vi "Build from database.vi"(8 "error in (no error)":errorcluster, 10 "Table Configuration":refnum<class "Table Configuration Interface.lvclass">, 11 "Table in":refnum<class "Basic Table.lvclass">) -> (0 "error out":errorcluster, 3 "Table out":refnum<class "Basic Table.lvclass">)   [LabVIEW 2020, in "Table.lvlib" / "Basic Table.lvclass"]
uses:
  Basic Table.lvclass
  Table Configuration Interface/Table Configuration Interface.lvclass
  Basic Table.lvclass/Basic Table.ctl
  Database Libraries/Database Interfaces/Primary Key Info.ctl
  Column Libraries/Basic Columns/Column Configuration/Basic Column Configuration Class/Column Configuration.lvclass
  Database Libraries/Database Interfaces/Database Interface Class/Database Interface.lvclass
  Column Libraries/Basic Columns/Column Configuration/Column Factory Parent Class/Column Factory.lvclass
  Database Libraries/Database Interfaces.lvlib
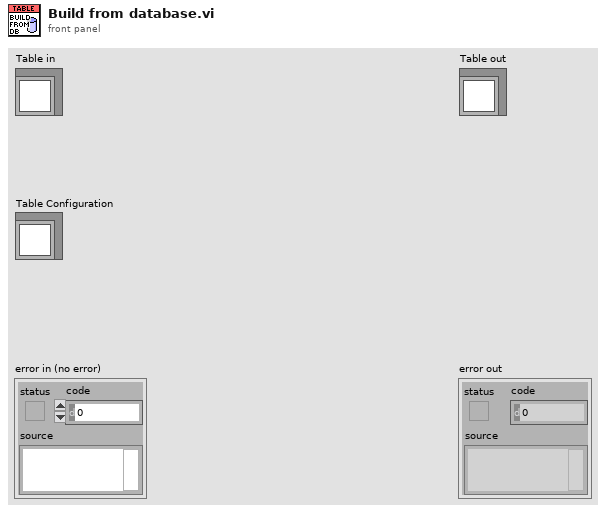
[diagram p1: front panel]
types:
  T1 = typedef "Database Interfaces.lvlib/Primary Key Info.ctl" = cluster{"Primary Key Column":string, "Display Column":string}
  T2 = typedef "Column Interfaces.lvlib/FK Info.ctl" = cluster{"PK Table":string, "PK Column":string, "PK Display Column":string}
  T3 = typedef "Database Interfaces.lvlib/Column Information.ctl" = cluster{"Name":string, "Type":T4, "Size (bytes)":i32}
  T4 = typedef "Database Interfaces.lvlib/Database data type.ctl" = enum16{"Undefined", "String", "Long (I32)", "Single (SGL)", "Double (DBL)", "Date/Time", "Binary"}
  T5 = map{string, refnum<class "Column Interface.lvclass">}
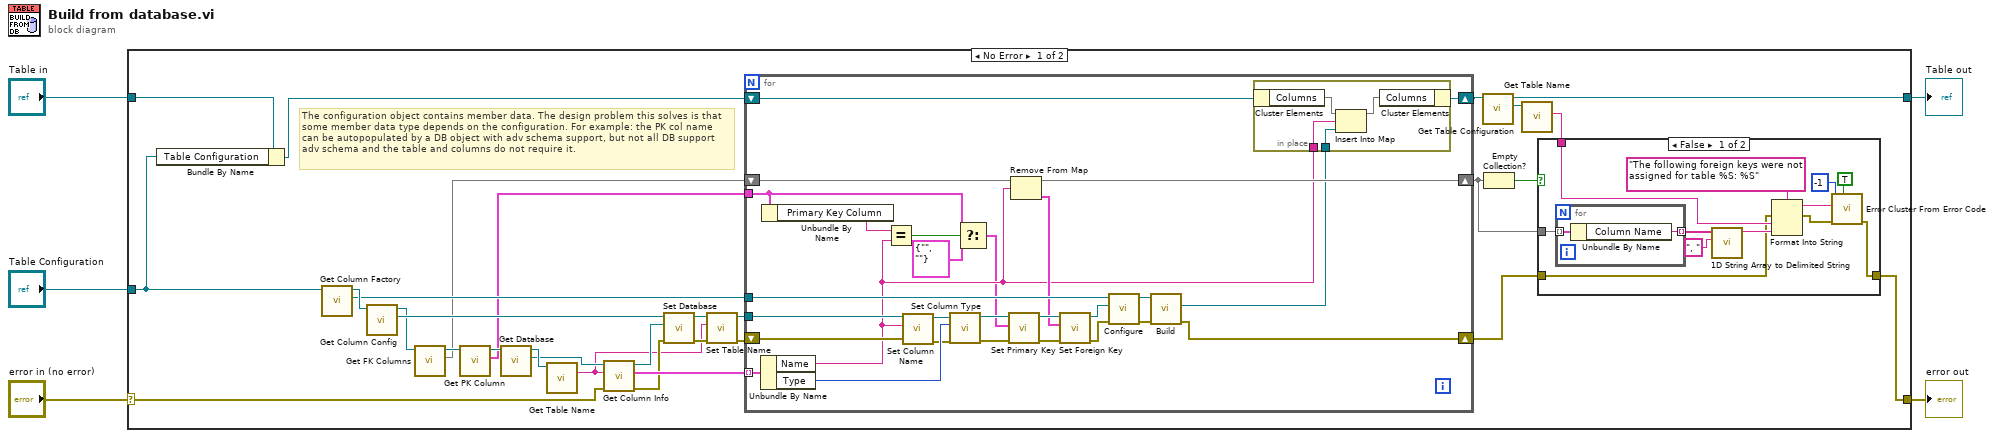
[diagram p0: block diagram]
diagram:
  n1 = case shown="No Error" "error in (no error)" {
    selector: "error in (no error)" -> [w29 w84]
    tunnel: [w7 w84] -> w4
    tunnel: [w10 w83] -> w2
    tunnel: "Table in" -> [w21 w83]
    tunnel: "Table Configuration" -> [w19 _]
    frame No Error {
      # "The configuration object contains member data. The design problem this solves is that some member data type depends on the configuration. For example: the PK col name can be autopopulated by a DB object with adv schema support, but not all DB support adv schema and the table and columns do not require it."
      n2 = Bundle By Name(cluster=w21, "Table Configuration"=w19) -> (w20:refnum<class "Basic Table.lvclass">)
      n3 = call-dynamic "Get Column Factory.vi"("Table Configuration Interface in"=w19) -> ("Column Factory"=w25:refnum<class "Column Factory.lvclass">, "Table Configuration Interface out"=w27:refnum<class "Table Configuration Interface.lvclass">)  [unwired: 8 in, 1 out]
      n4 = call-dynamic "Get Column Config.vi"("Table Configuration Interface in"=w27) -> ("Column Configuration"=w24:refnum<class "Column Configuration.lvclass">, "Table Configuration Interface out"=w18:refnum<class "Table Configuration Interface.lvclass">)  [unwired: 8 in, 1 out]
      n5 = call-dynamic "Get FK Columns.vi"("Table Configuration Interface in"=w18) -> ("FKs"=w15:map{string, T2}, "Table Configuration Interface out"=w17:refnum<class "Table Configuration Interface.lvclass">)  [unwired: 8 in, 1 out]
      n6 = call-dynamic "Get PK Column.vi"("Table Configuration Interface in"=w17) -> ("Primary Key"=w6:T1, "Table Configuration Interface out"=w16:refnum<class "Table Configuration Interface.lvclass">)  [unwired: 8 in, 1 out]
      n7 = call-dynamic "Get Database.vi"("Table Configuration Interface in"=w16) -> ("Database"=w23:refnum<class "Database Interface.lvclass">, "Table Configuration Interface out"=w26:refnum<class "Table Configuration Interface.lvclass">)  [unwired: 8 in, 1 out]
      n8 = call-dynamic "Get Table Name.vi"("Table Configuration Interface in"=w26) -> ("Table Name"=w22:string)  [unwired: 8 in, 2 out]
      n9 = call-dynamic "Get Column Info.vi"("error in (no error)"=w29, "Table Name"=w22, "Database Interface in"=w23) -> ("error out"=w32:errorcluster, "Column Information Array"=w35:T3[], "Database Interface out"=w28:refnum<class "Database Interface.lvclass">)  [unwired: 6 in]
      n10 = call-dynamic "Set Database.vi"("error in (no error)"=w32, "Database"=w28, "Basic Column Configuration in"=w24) -> ("error out"=w31:errorcluster, "Basic Column Configuration out"=w34:refnum<class "Column Configuration.lvclass">)  [unwired: 7 in]
      n11 = call-dynamic "Set Table Name.vi"("error in (no error)"=w31, "Table Name"=w22, "Basic Column Configuration in"=w34) -> ("error out"=w30:errorcluster, "Basic Column Configuration out"=w33:refnum<class "Column Configuration.lvclass">)  [unwired: 7 in]
      n12 = for {
        tunnel: w35 -> [w78] mode=indexing
        tunnel: w33 -> [w76]
        tunnel: w25 -> [w74]
        shift-right: [w71] -> w11
        shift-left: w20 -> [w72]
        shift-right: [w67] -> w12
        shift-left: w30 -> [w70]
        shift-right: [w59] -> w13
        shift-left: w15 -> [w60]
        tunnel: w6 -> [w55]
        n13 = Unbundle By Name(w78) -> ("Name"=w57:string, "Type"=w77:T4)
        n14 = Unbundle By Name(w55) -> ("Primary Key Column"=w56:string)
        n15 = Equal?(x=w56, y=w57) -> (x = y?=w52:bool)
        n16 = call-dynamic "Set Column Name.vi"("error in (no error)"=w70, "Column Name"=w57, "Basic Column Configuration in"=w76) -> ("error out"=w69:errorcluster, "Basic Column Configuration out"=w75:refnum<class "Column Configuration.lvclass">)  [unwired: 7 in]
        n17 = call-dynamic "Set Column Type.vi"("error in (no error)"=w69, "Column Type"=w77, "Basic Column Configuration in"=w75) -> ("error out"=w65:errorcluster, "Basic Column Configuration out"=w66:refnum<class "Column Configuration.lvclass">)  [unwired: 7 in]
        n18 = Select(t=w55, s=w52, f=T1 {"Primary Key Column"="", "Display Column"=""}) -> (s? t:f=w53:T1)
        n19 = call-dynamic "Set Primary Key.vi"("error in (no error)"=w65, "Primary Key"=w53, "Basic Column Configuration in"=w66) -> ("error out"=w63:errorcluster, "Basic Column Configuration out"=w64:refnum<class "Column Configuration.lvclass">)  [unwired: 7 in]
        n20 = Remove From Map(10:w57, 11:w60) -> (1:w58:T2, 3:w59:map{string, T2})  [unwired: 1 out]
        n21 = call-dynamic "Set Foreign Key.vi"("error in (no error)"=w63, "FK Info"=w58, "Basic Column Configuration in"=w64) -> ("error out"=w62:errorcluster, "Basic Column Configuration out"=w61:refnum<class "Column Configuration.lvclass">)  [unwired: 7 in]
        n22 = call-dynamic "Configure.vi"("error in (no error)"=w62, "Configuration"=w61, "Column Factory in"=w74) -> ("error out"=w68:errorcluster, "Column Factory out"=w73:refnum<class "Column Factory.lvclass">)  [unwired: 7 in]
        n23 = call-dynamic "Build.vi"("error in (no error)"=w68, "Column Factory in"=w73) -> ("error out"=w67:errorcluster, "Column"=w51:refnum<class "Column Interface.lvclass">)  [unwired: 7 in, 1 out]
        n24 = in-place {
          in-place-border: w51 -> [w80]
          in-place-border: w57 -> [w79]
          n25 = in-place-cluster #1(w72) -> ("Columns"=w82:T5)
          n26 = Insert Into Map(map in=w82, key=w79, value=w80) -> (map out=w81:T5)  [unwired: 2 out]
          n27 = in-place-cluster #1("Columns"=w81) -> (w71:refnum<class "Basic Table.lvclass">)
        }
      }
      n28 = call "Get Table Configuration.vi"("Basic Table in"=w11) -> ("Table Configuration"=w9:refnum<class "Table Configuration Interface.lvclass">, "Basic Table out"=w10:refnum<class "Basic Table.lvclass">)  [unwired: 8 in, 1 out]
      n29 = Empty Collection?(1:w13) -> (0:w14:bool)
      n30 = call-dynamic "Get Table Name.vi"("Table Configuration Interface in"=w9) -> ("Table Name"=w8:string)  [unwired: 8 in, 2 out]
      n31 = case shown="False" w14 {
        tunnel: w13 -> [w47 _]
        tunnel: w12 -> [w41 w50]
        tunnel: w8 -> [w42 _]
        tunnel: [w36 w50] -> w7
        frame False {
          n32 = for {
            tunnel: w47 -> [w49] mode=indexing
            tunnel: [w48] -> w46 mode=indexing
            n33 = Unbundle By Name(w49) -> ("Column Name"=w48:string)
          }
          n34 = call <vilib>:"1D String Array to Delimited String.vi"("delimiter"=", ", "string array"=w46) -> ("delimited string"=w43:string)  [unwired: 9 in]
          n35 = Format Into String(format string="The following foreign keys were not assigned for table %S: %S", error in=w41, w42, w43) -> (resulting string=w39:string, error out=w40:errorcluster)  [unwired: 1 in]
          n36 = call <vilib>:"Error Cluster From Error Code.vi"("show call chain? (False)"=TRUE, "error in (no error)"=w40, "error message (\"\")"=w39, "error code (0)"=-1) -> ("error out"=w36:errorcluster)  [unwired: 5 in]
        }
        frame True {
        }
      }
    }
    frame Error {
    }
  }
  "error out" <- w4
  "Table out" <- w2
